vi "Begin Transfer.vi"(8 "error in":errorcluster, 10 "SDO Transfer":refnum<class "SDO Transfer.lvclass">, 11 "Transfer Beginner in":refnum<class "Transfer Beginner.lvclass">) -> (0 "error out":errorcluster, 3 "Transfer Beginner out":refnum<class "Transfer Beginner.lvclass">)   [LabVIEW 2020, in "CANopen.lvlib" / "SDO Manager.lvlib" / "Transfer Beginner.lvlib" / "Transfer Beginner.lvclass"]
uses:
  Transfer Beginner.lvclass
  SDO Transfer/SDO Transfer.lvclass
  Transfer Beginner.lvclass/Transfer Beginner.ctl
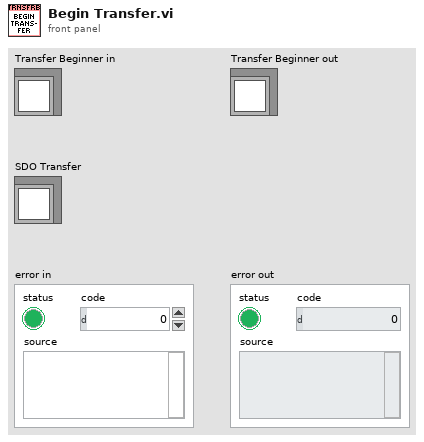
[diagram p1: front panel]
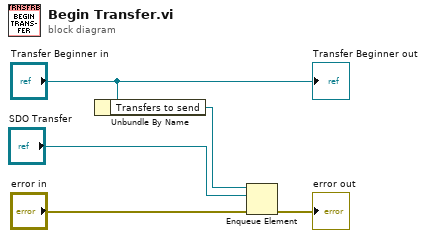
[diagram p0: block diagram]
diagram:
  n1 = Unbundle By Name("Transfer Beginner in") -> ("Transfers to send"=w2:refnum<queue>)
  n2 = Enqueue Element(queue=w2, element="SDO Transfer", error in (no error)="error in") -> (error out=→"error out":errorcluster)  [unwired: 1 in, 2 out]
  "Transfer Beginner out" <- "Transfer Beginner in"
